vi "FT10_Config Parse File.vi"(8 "error in (no error)":errorcluster, 10 "File Path Control":path=path "Config.ini") -> (0 "error out":errorcluster, 2 "Config cluster":T1={"Unitherm Port"="COM4", "Simulate Values"=TRUE})   [LabVIEW 2015]
uses:
  Controls/Control_Config Cluster.ctl
  Controls/Control_Config Unitherm Port.ctl
  Controls/Control_Config Simulate Values.ctl
  <vilib>/Utility/config.llb/Read Key (String).vi
  <vilib>/Utility/config.llb/NI_LVConfig.lvlib
panel:
  out "Unitherm value":string
  out "Simulation value":string="1"
  out "Simulation found?":bool=TRUE
  out "Unitherm found?":bool=TRUE
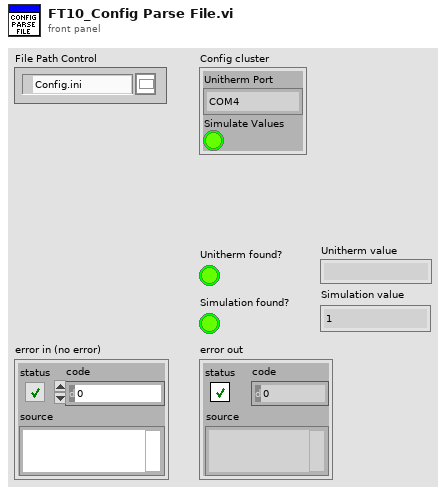
[diagram p1: front panel]
types:
  T1 = typedef "Control_Config Cluster.ctl" = cluster{"Unitherm Port":T2, "Simulate Values":T3}
  T2 = typedef "Control_Config Unitherm Port.ctl" = string
  T3 = typedef "Control_Config Simulate Values.ctl" = bool
  T4 = typedef "NI_LVConfig.lvlib/Config Data RefNum.ctl" = refnum<k1>
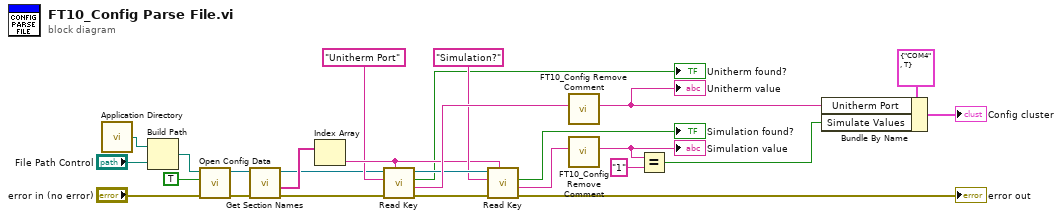
[diagram p0: block diagram]
diagram:
  n1 = call <vilib>:"Application Directory.vi"() -> ("Application Directory"=w5:path)
  n2 = Build Path(base path=w5, name or relative path="File Path Control") -> (appended path=w19:path)
  n3 = call <vilib>:"Open Config Data.vi"("error in (no error)"="error in (no error)", "create file if necessary (T)"=TRUE, "configuration file path"=w19) -> ("error out"=w4:errorcluster, "refnum"=w6:T4)  [unwired: 6 in, 1 out]
  n4 = call <vilib>:"Get Section Names.vi"("error in (no error)"=w4, "refnum"=w6) -> ("error out"=w8:errorcluster, "section names"=w10:string[], "refnum out"=w7:T4)  [unwired: 7 in]
  n5 = Index Array(array=w10) -> (element=w14:string)  [unwired: 1 in]
  n6 = call-poly <vilib>:"Read Key.vi"("section"=w14, "error in (no error)"=w8, "key"="Unitherm Port", "refnum"=w7) -> ("error out"=w12:errorcluster, "value"=w20:string, "found?"=→"Unitherm found?":bool, "refnum out"=w16:T4)  [unwired: 4 in]
  n7 = call-poly <vilib>:"Read Key.vi"("section"=w14, "error in (no error)"=w12, "key"="Simulation?", "refnum"=w16) -> ("error out"=→"error out":errorcluster, "value"=w21:string, "found?"=→"Simulation found?":bool)  [unwired: 4 in, 1 out]
  n8 = call "FT10_Config Remove Comment.vi"("Value In"=w20) -> ("Value without Comment"=w24:string)  [unwired: 10 in]
  "Unitherm value" <- w24
  n9 = call "FT10_Config Remove Comment.vi"("Value In"=w21) -> ("Value without Comment"=w22:string)  [unwired: 10 in]
  "Simulation value" <- w22
  n10 = Equal?(x=w22, y="1") -> (x = y?=w25:bool)
  n11 = Bundle By Name(cluster=T1 {"Unitherm Port"="COM4", "Simulate Values"=TRUE}, "Unitherm Port"=w24, "Simulate Values"=w25) -> (→"Config cluster":T1)
